vi "IO_18v7Send.vi"(8 "error in (no error)":errorcluster, 10 "Tx Buf Out":string, 11 "VISA Refnum in":refnum<visa-resource-name>) -> (0 "error out":errorcluster, 2 "read buffer":string, 3 "VISA Refnum out":refnum<visa-resource-name>)   [LabVIEW 2024]
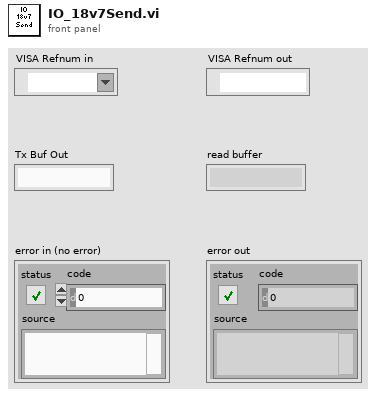
[diagram p1: front panel]
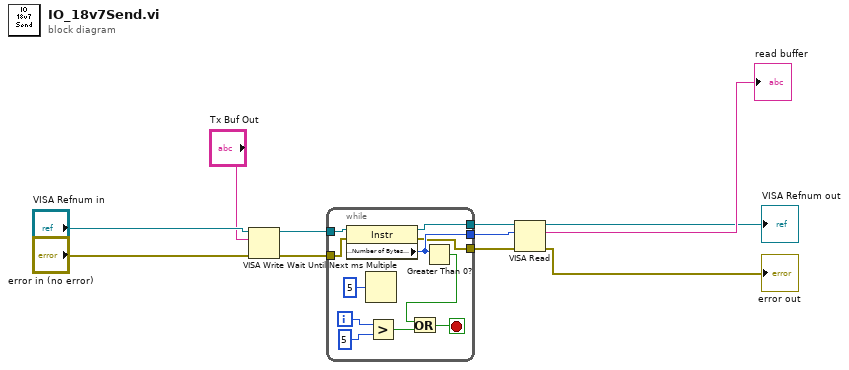
[diagram p0: block diagram]
diagram:
  n1 = VISA Write(VISA resource name="VISA Refnum in", write buffer="Tx Buf Out", error in (no error)="error in (no error)") -> (VISA resource name out=w3:refnum<visa-resource-name>, error out=w9:errorcluster)  [unwired: 1 out]
  n2 = while {
    tunnel: w3 -> [w21]
    tunnel: [w15] -> w4
    tunnel: [w14] -> w5
    tunnel: w9 -> [w13]
    tunnel: [w12] -> w10
    i -> [w18]
    stop <- w20 stop-if-true
    n3 = property class="Instr"(reference=w21, error in=w13) -> (reference out=w15:refnum<visa-resource-name>, error out=w12:errorcluster, "Serial Settings:Number of Bytes at Serial Port"=w14:u32)
    n4 = Wait Until Next ms Multiple(millisecond multiple=u32 5) -> ()  [unwired: 1 out]
    n5 = Greater?(x=w18, y=5) -> (0:w19:bool)
    n6 = Greater Than 0?(x=w14) -> (x > 0?=w16:bool)
    n7 = Or(x=w16, y=w19) -> (x .or. y?=w20:bool)
  }
  n8 = VISA Read(VISA resource name=w4, byte count=w5, error in (no error)=w10) -> (VISA resource name out=→"VISA Refnum out":refnum<visa-resource-name>, read buffer=→"read buffer":string, error out=→"error out":errorcluster)  [unwired: 1 out]
